vi "crio_subvi_encoder.vi"(4 "32 bit in":i32, 6 "Position Reset":bool, 7 "Debug: ConnectorA/DIO15":bool, 9 "Debug: ConnectorA/DIO14 2":bool, 10 "Debug: ConnectorA/DIO14":bool, 11 "Debug: ConnectorA/DIO15 2":bool) -> (3 "32 bit out":i32)   [LabVIEW 2019]
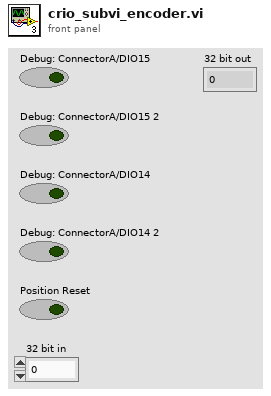
[diagram p1: front panel]
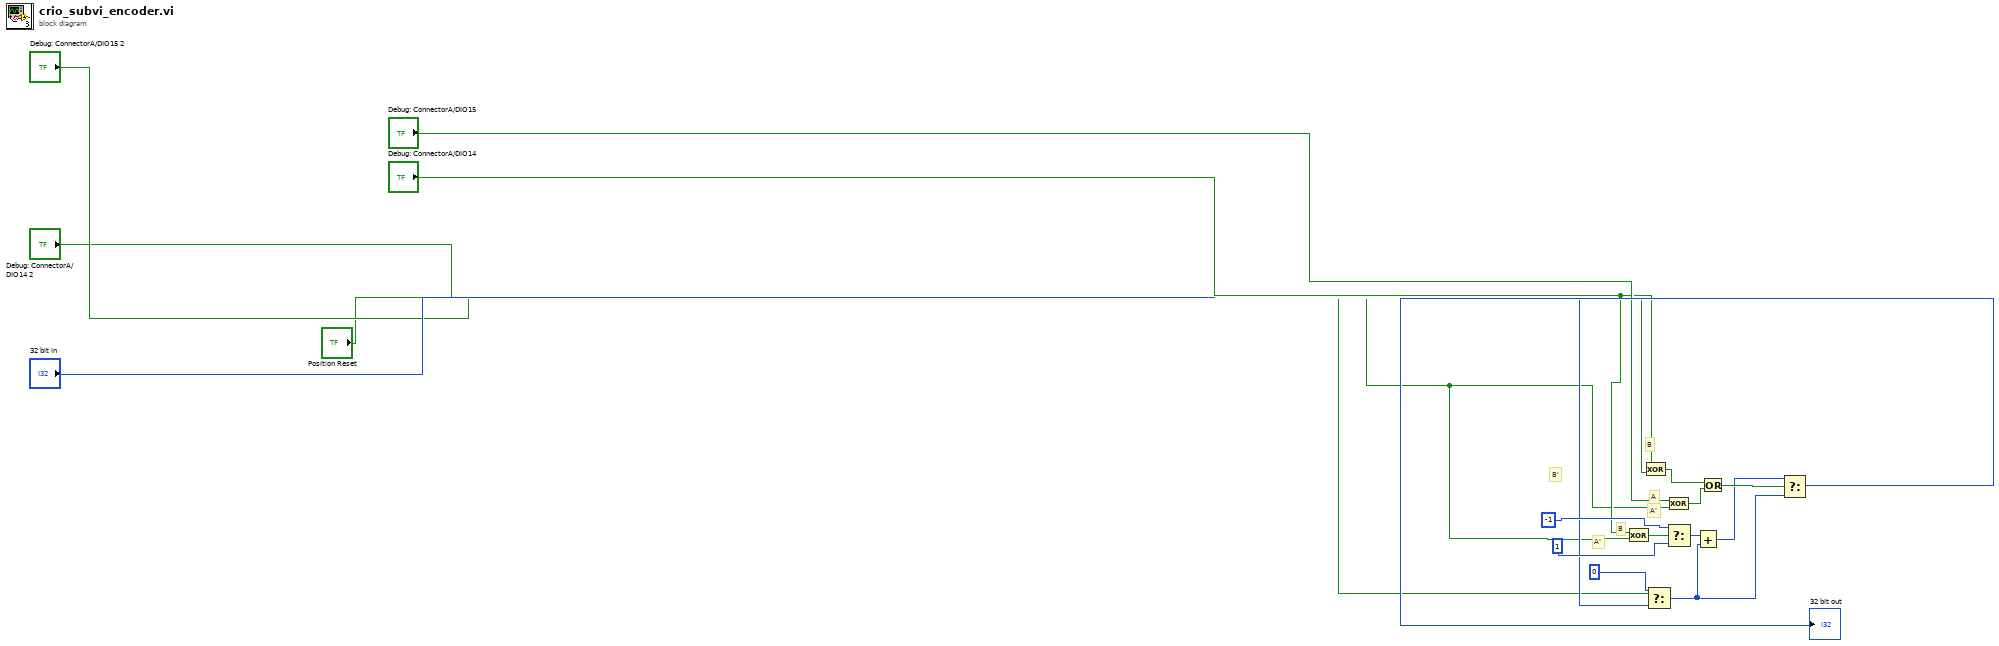
[diagram p0: block diagram]
diagram:
  # "B'"
  # "A'"
  # "B"
  # "A'"
  # "A"
  # "B"
  n1 = Exclusive Or(1:"Debug: ConnectorA/DIO15 2", 2:"Debug: ConnectorA/DIO14") -> (0:w16:bool)
  n2 = Exclusive Or(1:"Debug: ConnectorA/DIO14 2", 2:"Debug: ConnectorA/DIO14") -> (0:w15:bool)
  n3 = Select(t=0 ("32 bit"), s="Position Reset", f="32 bit in") -> (s? t:f=w10:i32)
  n4 = Exclusive Or(1:"Debug: ConnectorA/DIO15 2", 2:"Debug: ConnectorA/DIO15") -> (0:w14:bool)
  n5 = Select(t=-1 ("32 bit"), s=w16, f=1 ("32 bit")) -> (s? t:f=w11:i32)
  n6 = Add(x=w11, y=w10) -> (x+y=w8:i32)
  n7 = Or(x=w15, y=w14) -> (x .or. y?=w17:bool)
  n8 = Select(t=w8, s=w17, f=w10) -> (s? t:f=→"32 bit out":i32)
